vi "Barcode(SN)_Check.vi"(7 "Information":refnum<vi>, 10 "Limit":string) -> (2 "TestResult":bool, 3 "TestData":string, 5 "Information":refnum<vi>)   [LabVIEW 2013]
uses:
  MainProgram/Control/Buffer.vi
  <vilib>/Utility/config.llb/NI_LVConfig.lvlib
  <vilib>/Utility/config.llb/Read Key (String).vi
panel:
  out "Array":string[](array[string])
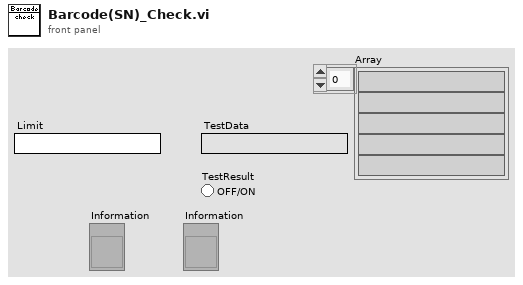
[diagram p1: front panel]
types:
  T1 = typedef "NI_LVConfig.lvlib/Config Data RefNum.ctl" = refnum<k1>
  T2 = typedef "StatusInformation.ctl" = cluster{"FileName:":string, "Barcode(S/N):":string, "TestStep:":string, "TestTime:":string, "Station:":string, "Model:":string, "Line:":string, "Status:":string, "Series:":string, "Reserve:":string}
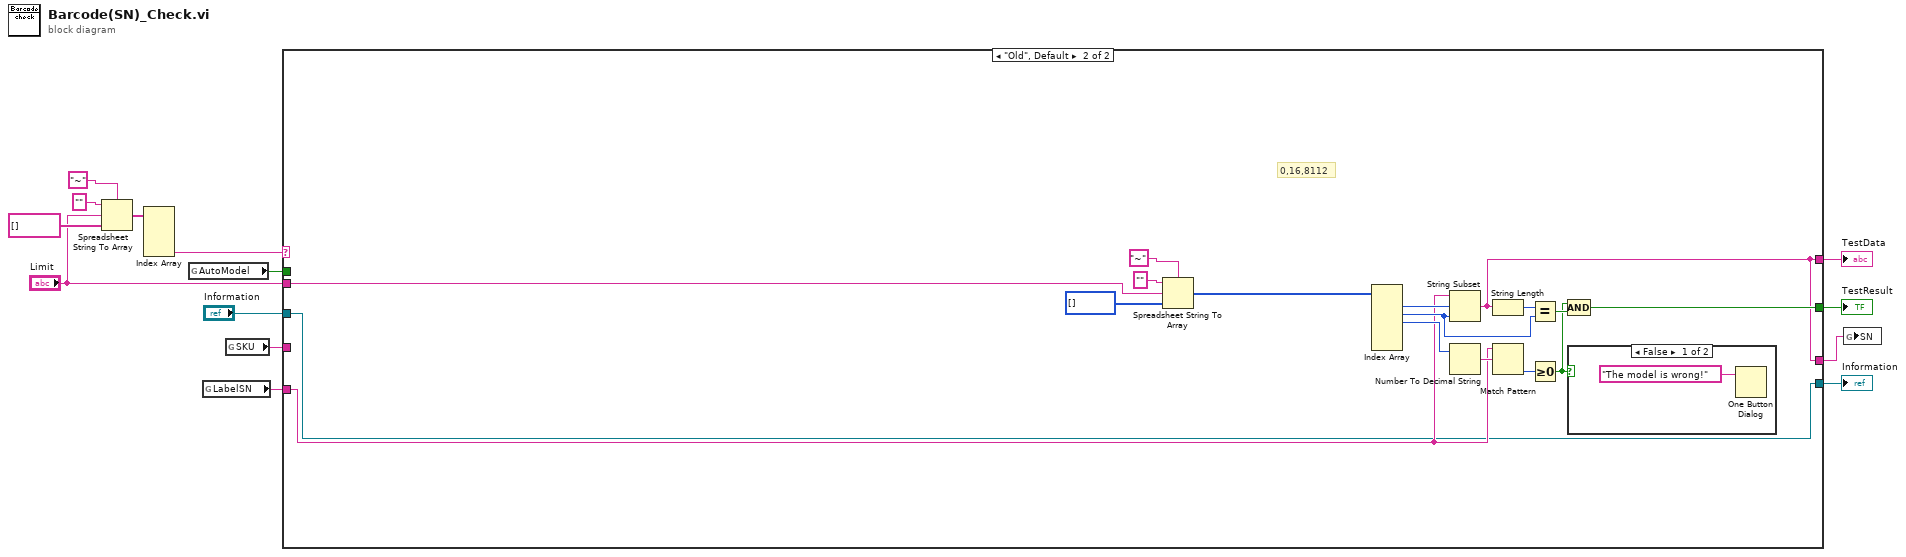
[diagram p0: block diagram]
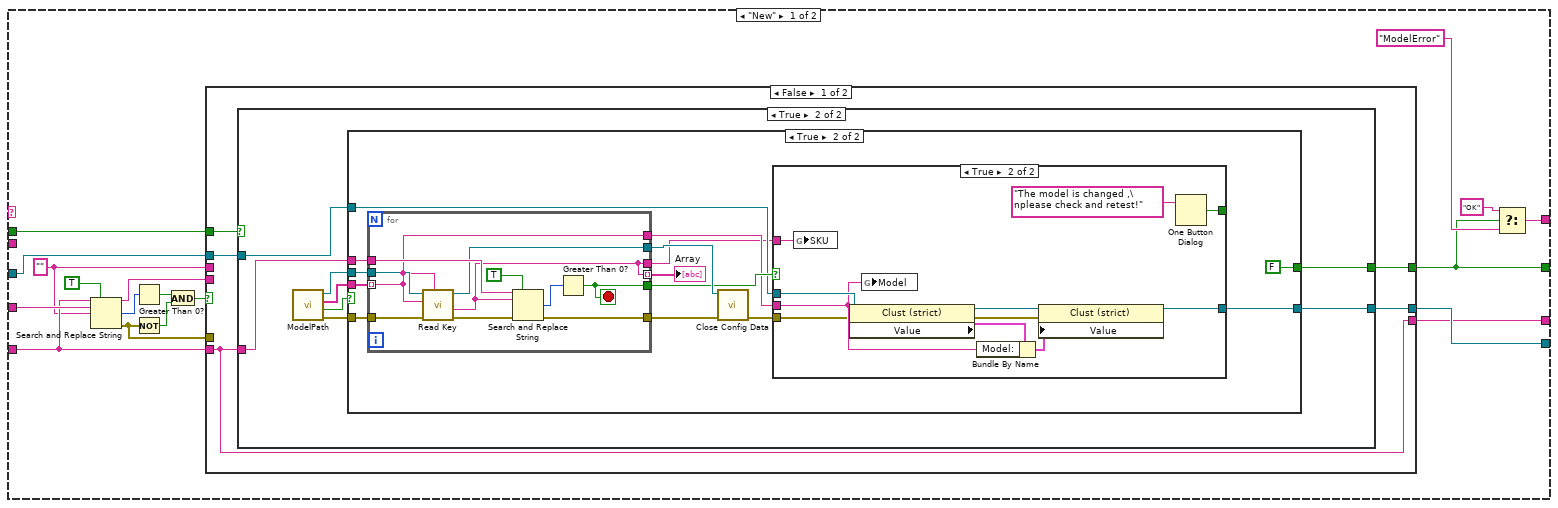
[diagram p2: hidden frame]
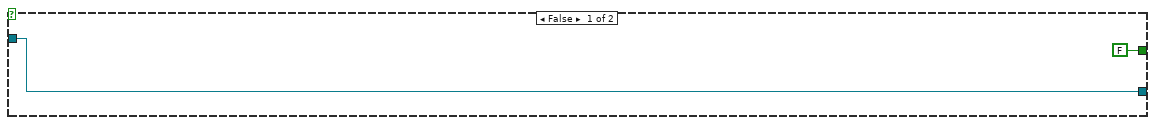
[diagram p3: hidden frame]
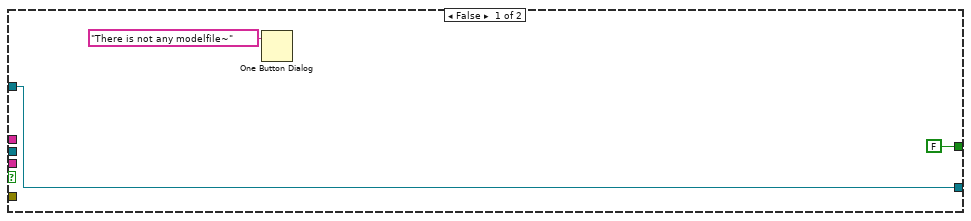
[diagram p4: hidden frame]
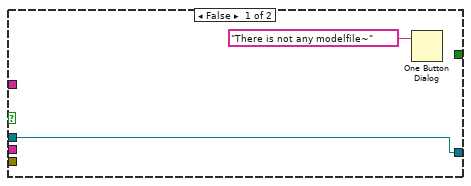
[diagram p5: hidden frame]
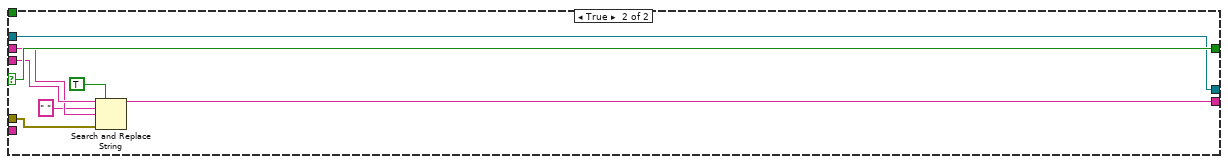
[diagram p6: hidden frame]
diagram:
  n1 = Spreadsheet String To Array(delimiter (Tab)="~", format string="", spreadsheet string="Limit", array type (2D Dbl)=string[] []) -> (array=w9:string[])
  n2 = Index Array(array=w9) -> (element #4=w8:string)  [unwired: 4 in, 3 out]
  n3 = global read "Buffer.vi" "AutoModel"() -> (w1:bool)
  n4 = global read "Buffer.vi" "LabelSN"() -> (w7:string)
  n5 = global read "Buffer.vi" "SKU"() -> (w4:string)
  n6 = case shown="\"Old\", Default" w8 {
    tunnel: "Limit" -> [_ w110]
    tunnel: [w19 w104] -> w14
    tunnel: w7 -> [w25 w100]
    tunnel: [w17 w99] -> w6
    tunnel: [w28 w99] -> w5
    tunnel: w4 -> [w32 _]
    tunnel: "Information" -> [w30 w97]
    tunnel: [w29 w97] -> w2
    tunnel: w1 -> [w20 _]
    frame "New" {
      w15 = "" ("replace string (\"\")")
      n7 = Search and Replace String(replace all?=TRUE ("replace all? (F)"), input string=w25, search string=w32, replace string=w15) -> (result string=w18:string, number of replacements=w31:i32, error out=w16:errorcluster)  [unwired: 4 in, 1 out]
      n8 = Greater Than 0?(x=w31) -> (x > 0?=w24:bool)
      n9 = Not(x=w16) -> (.not. x?=w23:bool)
      n10 = And(x=w24, y=w23) -> (x .and. y?=w22:bool)
      n11 = case shown="False" w22 {
        selector: w22 -> [_ w96]
        tunnel: w30 -> [w37 w95]
        tunnel: [w36 w95] -> w29
        tunnel: w25 -> [w33 _]
        tunnel: [w35 w96] -> w19
        tunnel: w20 -> [w34 _]
        tunnel: [w33 w93] -> w17
        tunnel: w18 -> [_ w94]
        tunnel: w16 -> [_ w92]
        tunnel: w15 -> [_ w91]
        frame False {
          n12 = case shown="True" w34 {
            tunnel: w37 -> [w39 w41]
            tunnel: [w39 w40] -> w36
            tunnel: w33 -> [_ w45]
            tunnel: [FALSE w44] -> w35
            frame False {
            }
            frame True {
              n13 = call "ModelPath.vi"() -> ("error out"=w43:errorcluster, "found?"=w42:bool, "Models"=w47:string[], "Refnum out"=w46:T1)  [unwired: 8 in]
              n14 = case shown="True" w42 {
                tunnel: w47 -> [_ w64]
                tunnel: w46 -> [_ w63]
                tunnel: w45 -> [_ w53]
                tunnel: [FALSE FALSE] -> w44
                tunnel: w43 -> [_ w60]
                tunnel: w41 -> [w48 w57]
                tunnel: [w48 w56] -> w40
                frame False {
                  n15 = One Button Dialog(message="There is not any modelfile~") -> ()  [unwired: 1 in, 1 out]
                }
                frame True {
                  n16 = for {
                    tunnel: w64 -> [w85] mode=indexing
                    tunnel: w63 -> [w88]
                    tunnel: w53 -> [w87]
                    tunnel: [w79] -> w55
                    tunnel: [w85] -> w58
                    tunnel: [w84] -> w59
                    tunnel: [w83] -> w62
                    tunnel: [w81] -> w61
                    tunnel: w60 -> [w80]
                    tunnel: [w79] -> w54 mode=indexing
                    stop <- w84 stop-if-true
                    n17 = call-poly <vilib>:"Read Key.vi"("section"=w85, "error in (no error)"=w80, "key"=w85, "refnum"=w88) -> ("error out"=w82:errorcluster, "value"=w79:string, "refnum out"=w83:T1)  [unwired: 4 in, 1 out]
                    n18 = Search and Replace String(replace all?=TRUE ("replace all? (F)"), input string=w87, search string=w79, error in=w82) -> (number of replacements=w86:i32, error out=w81:errorcluster)  [unwired: 4 in, 2 out]
                    n19 = Greater Than 0?(x=w86) -> (x > 0?=w84:bool)
                  }
                  "Array" <- w54
                  n20 = call <vilib>:"Close Config Data.vi"("error in (no error)"=w61, "refnum"=w62) -> ("error out"=w52:errorcluster)  [unwired: 8 in, 1 out]
                  n21 = case shown="True" w59 {
                    tunnel: w57 -> [w66 w73]
                    tunnel: [w66 w72] -> w56
                    tunnel: w58 -> [_ w71]
                    tunnel: w55 -> [_ w70]
                    tunnel: w52 -> [_ w67]
                    tunnel: [_ w69] -> _
                    frame False {
                      n22 = One Button Dialog(message="There is not any modelfile~") -> ()  [unwired: 1 in, 1 out]
                    }
                    frame True {
                      n23 = global write "Buffer.vi" "SKU"(w70) -> ()
                      n24 = property class="Clust (strict)"(reference=w73, error in=w67) -> (reference out=w75:refnum<vi>, error out=w77:errorcluster, "Value"=w76:T2)
                      n25 = global write "Buffer.vi" "Model"(w71) -> ()
                      n26 = Bundle By Name(cluster=w76, "Model:"=w71) -> (w74:T2)
                      n27 = property class="Clust (strict)"(reference=w75, error in=w77, "Value"=w74) -> (reference out=w72:refnum<vi>)  [unwired: 1 out]
                      n28 = One Button Dialog(message="The model is changed ,\nplease check and retest!") -> (true=w69:bool)  [unwired: 1 in]
                    }
                  }
                }
              }
            }
          }
        }
        frame True {
          n29 = Search and Replace String(replace all?=TRUE ("replace all? (F)"), input string=w94, search string=" ", replace string=w91, error in=w92) -> (result string=w93:string)  [unwired: 3 in, 3 out]
        }
      }
      n30 = Select(t="OK", s=w19, f="ModelError") -> (s? t:f=w28:string)
    }
    frame "Old", Default {
      # "0,16,8112"
      n31 = Spreadsheet String To Array(delimiter (Tab)="~", format string="", spreadsheet string=w110, array type (2D Dbl)=i32[] []) -> (array=w109:i32[])
      n32 = Index Array(array=w109) -> (element #1=w108:i32, element #2=w106:i32, element #3=w103:i32)  [unwired: 6 in, 3 out]
      n33 = String Subset(string=w100, offset (0)=w108, length (rest)=w106) -> (substring=w99:string)
      n34 = Number To Decimal String(number=w103) -> (decimal integer string=w102:string)  [unwired: 1 in]
      n35 = String Length(string=w99) -> (length=w107:i32)
      n36 = Match Pattern(string=w100, regular expression=w102) -> (offset past match=w101:i32)  [unwired: 1 in, 3 out]
      n37 = Equal?(x=w107, y=w106) -> (x = y?=w105:bool)
      n38 = Greater Or Equal To 0?(x=w101) -> (x >= 0?=w98:bool)
      n39 = Compound Arithmetic op=AND(w98, w105) -> (w104:bool)
      n40 = case shown="False" w98 {
        frame False {
          n41 = One Button Dialog(message="The model is wrong!") -> ()  [unwired: 1 in, 1 out]
        }
        frame True {
        }
      }
    }
  }
  "TestResult" <- w14
  "TestData" <- w5
  "Information" <- w2
  n42 = global write "Buffer.vi" "SN"(w6) -> ()
